vi "Create Virtual Axis.vi"   [LabVIEW 2018, in "Zaber A Series.lvlib"]
uses:
  Zaber A Series.lvlib
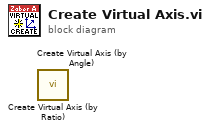
[diagram p0: block diagram]
diagram:
  n1 = call "Create Virtual Axis (by Ratio).vi"() -> ()  [unwired: 10 in, 2 out]
  n2 = call "Create Virtual Axis (by Angle).vi"() -> ()  [unwired: 10 in, 2 out]
